vi "Write channel pointer.vi"(8 "error in (no error)":errorcluster, 10 "channel pointer":u64 format="%.0x", 11 "Class 2 in":refnum<class "Class 2345678.lvclass">) -> (0 "error out":errorcluster, 3 "Class 2 out":refnum<class "Class 2345678.lvclass">)   [LabVIEW 2016, in "Data Sharing Framework.Runtime.lvlib" / "Class 2345678.lvclass"]
uses:
  Class 2345678.lvclass
  Class 2345678.lvclass/Class 2345678.ctl
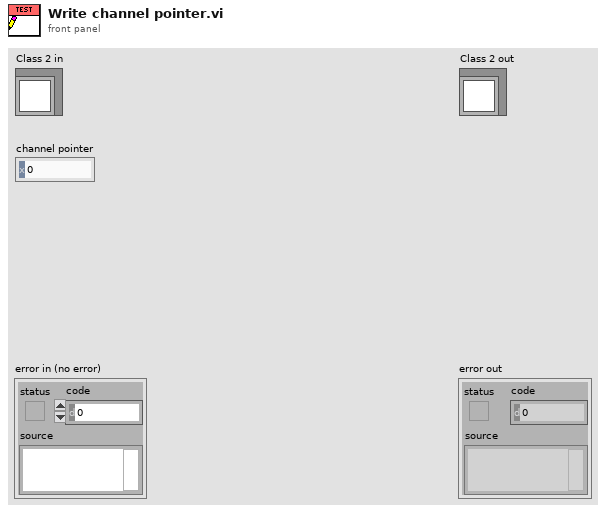
[diagram p1: front panel]
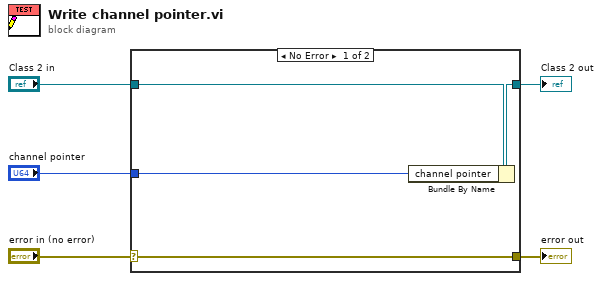
[diagram p0: block diagram]
diagram:
  n1 = case shown="No Error" "error in (no error)" {
    selector: "error in (no error)" -> [w9 w10]
    tunnel: [w9 w10] -> w4
    tunnel: [w7 w11] -> w2
    tunnel: "Class 2 in" -> [w8 w11]
    tunnel: "channel pointer" -> [w6 _]
    frame No Error {
      n2 = Bundle By Name(cluster=w8, "channel pointer"=w6) -> (w7:refnum<class "Class 2345678.lvclass">)
    }
    frame Error {
    }
  }
  "error out" <- w4
  "Class 2 out" <- w2
